vi "Cleanup Block Diagram.vi"(8 "error in (no error)":errorcluster, 10 "Clean Up Options":T1={"Alignment"=enum."Gravity", "Rules"=enum."Allow Wires Under Wide Blocks", "Max Heuristic Iterations"=200, "Max Simplex Iterations"=200, "Block Padding"={"Horizontal"=50, "Vertical"=50}, "Wire Padding"={"Horizontal"=10, "Vertical"=10}, "Auto-Tune by Topology"=TRUE, "Fine-Tune Y Positions"=TRUE, "Align All Controls on Left"=TRUE, "Align All Indicators on Right"=TRUE, "Use Array Dimension Heuristics"=FALSE}, 11 "VI Path":path) -> (0 "error out":errorcluster, 3 "VI Path Out":path)   [LabVIEW 2016, in "SLL Scripting.lvlib" / "SLL Class DVR API Generator.lvlib"]
uses:
  SLL Class DVR API Generator.lvlib
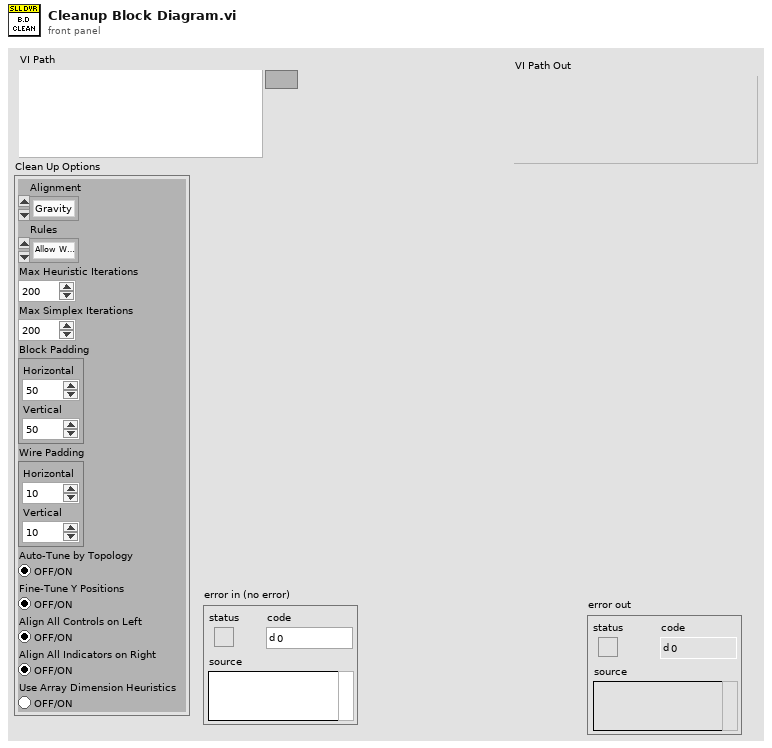
[diagram p1: front panel]
types:
  T1 = cluster{"Alignment":enum32{"Left", "Right", "Hybrid", "Center", "Gravity"}, "Rules":enum32{"Strict", "Allow Wires Under Labels", "Allow Wires Under Lead Nodes", "Allow Wires Under Wide Blocks"}, "Max Heuristic Iterations":u32, "Max Simplex Iterations":u32, "Block Padding":cluster{"Horizontal":i32, "Vertical":i32}, "Wire Padding":cluster{"Horizontal":i32, "Vertical":i32}, "Auto-Tune by Topology":bool, "Fine-Tune Y Positions":bool, "Align All Controls on Left":bool, "Align All Indicators on Right":bool, "Use Array Dimension Heuristics":bool}
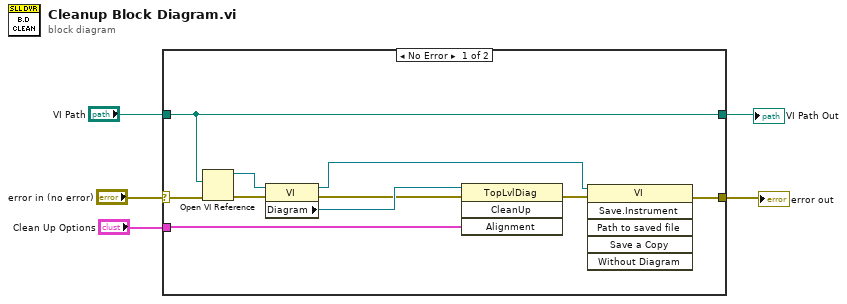
[diagram p0: block diagram]
diagram:
  n1 = case shown="No Error" "error in (no error)" {
    selector: "error in (no error)" -> [w15 w17]
    tunnel: [w10 w17] -> w4
    tunnel: "VI Path" -> [w12 w16]
    tunnel: [w12 w16] -> w1
    tunnel: "Clean Up Options" -> [w6 _]
    frame No Error {
      n2 = Open VI Reference(vi path=w12, error in (no error)=w15) -> (vi reference=w13:refnum<vi>, error out=w14:errorcluster)  [unwired: 4 in]
      n3 = property class="VI"(reference=w13, error in=w14) -> (reference out=w9:refnum<vi>, error out=w8:errorcluster, "Diagram"=w11:refnum<vi>)
      n4 = invoke class="TopLvlDiag" method="CleanUp"(reference=w11, error in=w8, "Alignment"=w6) -> (error out=w7:errorcluster)  [unwired: 1 in, 3 out]
      n5 = invoke class="VI" method="Save.Instrument"(reference=w9, error in=w7) -> (error out=w10:errorcluster)  [unwired: 4 in, 5 out]
    }
    frame Error {
    }
  }
  "error out" <- w4
  "VI Path Out" <- w1
